vi "Do.vi"(8 "error in (no error)":errorcluster, 10 "Actor in":refnum<class "Actor.lvclass">, 11 "StartTask Msg":refnum<class "StartTask Msg.lvclass">) -> (0 "error out":errorcluster, 2 "Actor out":refnum<class "Actor.lvclass">)   [LabVIEW 2025, in "Task_Abstr.lvlib" / "StartTask Msg.lvclass"]
doc: "This VI delivers the message to the actor by calling the appropriate method(s) on the actor."
uses:
  StartTask Msg.lvclass
  <vilib>/ActorFramework/Actor/Actor.lvclass
  Task_Abstr/Task_Abstr.lvclass
  5bf83c0c-2b59-4de7-a1cb-f3213895891a.vi
  StartTask Msg.lvclass/StartTask Msg.ctl
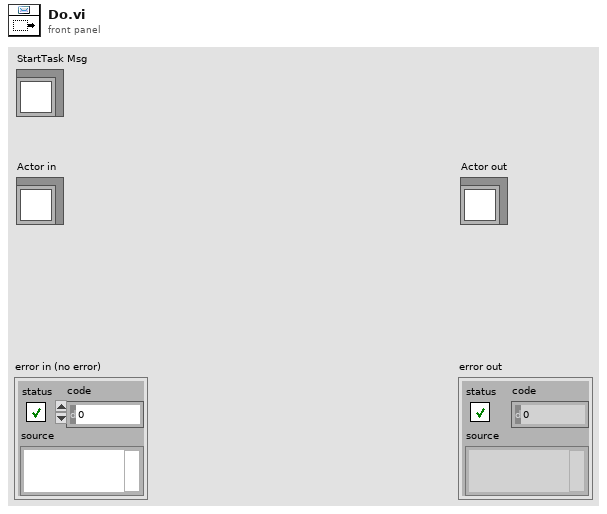
[diagram p1: front panel]
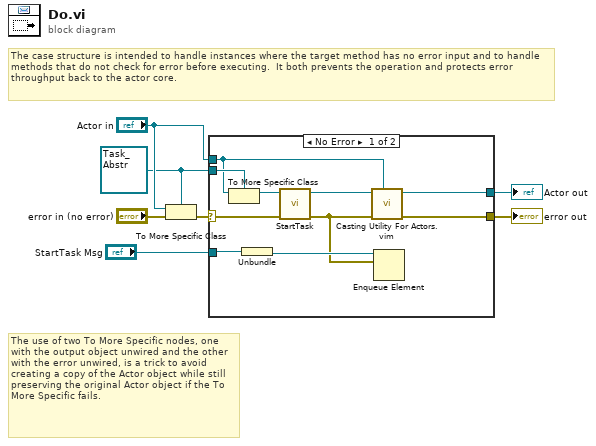
[diagram p0: block diagram]
diagram:
  w3 = refnum<class "Task_Abstr.lvclass"> refnum ("Actor in")
  # "The use of two To More Specific nodes, one with the output object unwired and the other with the error unwired, is a trick to avoid creating a copy of the Actor object while still preserving the original Actor object if the To More Specific fails."
  # "The case structure is intended to handle instances where the target method has no error input and to handle methods that do not check for error before executing.  It both prevents the operation and protects error throughput back to the actor core."
  n1 = To More Specific Class(target class=w3, reference="Actor in", error in="error in (no error)") -> (error out=w2:errorcluster)  [unwired: 1 out]
  n2 = case shown="No Error" w2 {
    selector: w2 -> [w17 w19]
    tunnel: [w11 w19] -> w7
    tunnel: [w12 w18] -> w6
    tunnel: "Actor in" -> [w14 w18]
    tunnel: w3 -> [w15 _]
    tunnel: "StartTask Msg" -> [w10 _]
    frame No Error {
      n3 = To More Specific Class(target class=w15, reference=w14) -> (specific class reference=w16:refnum<class "Task_Abstr.lvclass">)  [unwired: 1 in, 1 out]
      n4 = Unbundle(w10) -> (w9:refnum<queue>)
      n5 = call-dynamic "StartTask.vi"("error in (no error)"=w17, "Task_Abstr in"=w16) -> ("error out"=w8:errorcluster, "Task_Abstr out"=w13:refnum<class "Task_Abstr.lvclass">)  [unwired: 8 in]
      n6 = call "Casting Utility For Actors.vim"("type"=w14, "error in (no error)"=w8, "Actor in"=w13) -> ("error out"=w11:errorcluster, "Actor out"=w12:refnum<class "Actor.lvclass">)  [unwired: 7 in]
      n7 = Enqueue Element(queue=w9, element=w8) -> ()  [unwired: 2 in, 3 out]
    }
    frame Error {
      # "If type check fails, pass the original object out again."
    }
  }
  "error out" <- w7
  "Actor out" <- w6
